vi "Set Sensor Params Array.vi"(10 "SensorCfgParams Array":T1[](array[typedef]) {"CalibrCoefArray" format="%#.12g"}, 11 "Select Probe":i32) -> ()   [LabVIEW 2015, in "Tool Cfg.lvlib"]
uses:
  Tool Cfg.lvlib
  _SensorConfigParams Cluster--typedef.ctl
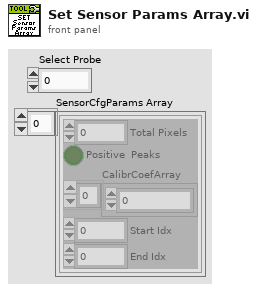
[diagram p1: front panel]
types:
  T1 = typedef "Tool Cfg.lvlib/_SensorConfigParams Cluster--typedef.ctl" = cluster{"Total Pixels":u16, "Positive  Peaks":bool, "CalibrCoefArray":dbl[], "Start Idx":u16, "End Idx":u16}
  T2 = typedef "Tool Cfg.lvlib/_Sensor Block Cluster--typedef.ctl" = cluster{"nSensors":u16, "SensorCfgParams Array":T1[]}
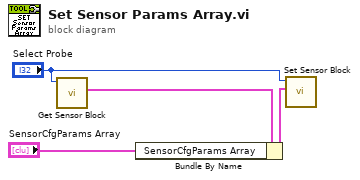
[diagram p0: block diagram]
diagram:
  n1 = call "Get Sensor Block.vi"("Select Probe"="Select Probe") -> ("Sensor Block"=w4:T2)  [unwired: 10 in]
  n2 = Bundle By Name(cluster=w4, "SensorCfgParams Array"="SensorCfgParams Array") -> (w2:T2)
  n3 = call "Set Sensor Block.vi"("Sensor Block"=w2, "Select Probe"="Select Probe") -> ()  [unwired: 10 in]
